vi "ReadinifileOutAllStr.vi"(8 "error in (no error)":errorcluster caption="错误输入（无错误）", 11 "appended path":path) -> (0 "error out":errorcluster caption="错误输出", 3 "字符串":string)   [LabVIEW 2018]
panel:
  # "E:\\2222222222222222222\\ATE_Program20201104\\ModelInformation\\test.ini"
  # "F:\\2222222222222222222\\ATE_Program20201104\\ModelInformation\\Eggy 55W.ini"
  # "E:\\2222222222222222222\\ATE_Program20201104\\ModelInformation\\Eggy 55W.ini"
  # "C:\\Users\\Administrator\\Desktop\\变压器FM9516_01\\FM9516\\ATE_Program20201123\\ModelInformation\\WHALE120W.ini"
  # "C:\\Users\\XCY\\Desktop\\变压器FM9516_01\\FM9516\\ATE_Program20210615\\ModelInformation"
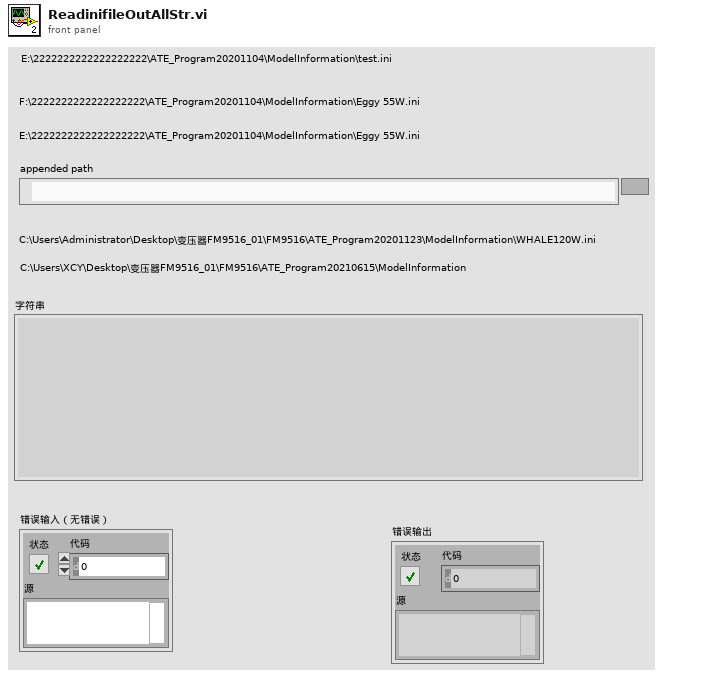
[diagram p1: front panel]
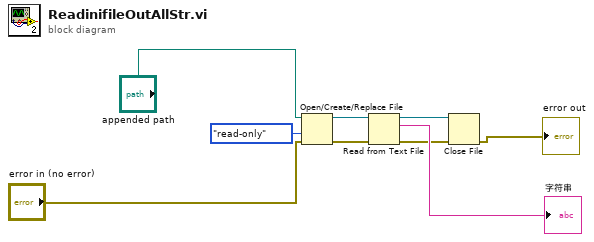
[diagram p0: block diagram]
diagram:
  n1 = Open/Create/Replace File(file path (use dialog)="appended path", error in="error in (no error)", access (0:read/write)=enum16{"read/write", "read-only", "write-only"}."read-only" ("权限(0:read/write)")) -> (refnum out=w7:refnum<file>, error out=w3:errorcluster)  [unwired: 3 in, 1 out]
  n2 = Read from Text File(file (use dialog)=w7, error in=w3) -> (refnum out=w8:refnum<file>, text=→"字符串":string, error out=w2:errorcluster)  [unwired: 2 in, 1 out]
  n3 = Close File(refnum=w8, error in=w2) -> (error out=→"error out":errorcluster)  [unwired: 1 out]
